vi "Advanced Params.vi"(6 "ID (Profile)":string="Profile", 7 "ADV params":T1={"ID"="", "Units"=enum."Metric", "RefPos"=0.0, "Cycles"=1, "Steps"=1, "Autoreturn"=FALSE, "BreakStop"=FALSE} {"Steps" min=1 max=12 step=1; "Cycles" min=1 max=60000 step=1}, 8 "error in (no error)":errorcluster, 11 "Profile NO":u8=1 min=1 max=50 step=1) -> (0 "error out":errorcluster, 2 "wchitch params":string, 3 "params array out":string[](array[string]))   [LabVIEW 2019, in "STAV lib.lvlib"]
uses:
  STAV lib.lvlib
  Advanced prams.ctl
  Param Units.ctl
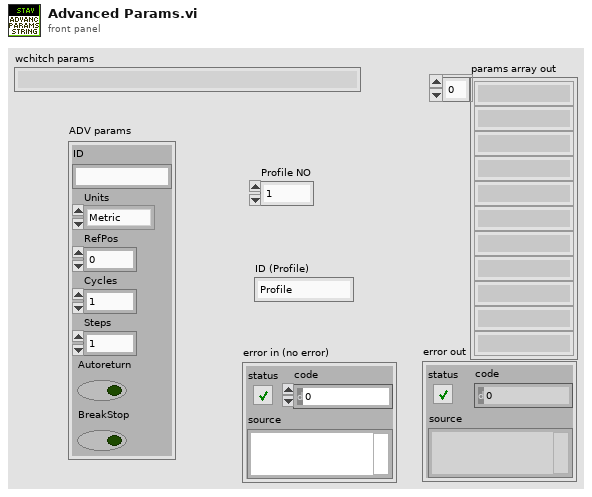
[diagram p1: front panel]
types:
  T1 = typedef "STAV lib.lvlib/Advanced prams.ctl" = cluster{"ID":string, "Units":T2, "RefPos":dbl, "Cycles":i32, "Steps":i32, "Autoreturn":bool, "BreakStop":bool}
  T2 = typedef "STAV lib.lvlib/Param Units.ctl" = enum16{"Metric", "Imperial"}
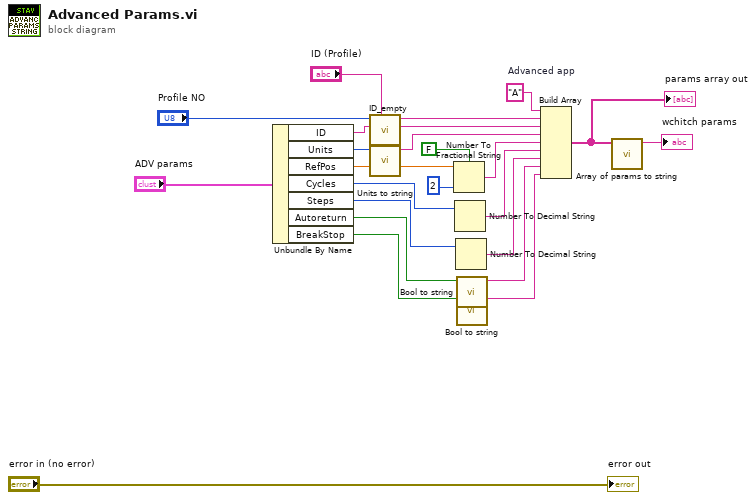
[diagram p0: block diagram]
diagram:
  w24 = "A"  # Advanced app
  n1 = Unbundle By Name("ADV params") -> ("ID"=w14:string, "Units"=w21:T2, "RefPos"=w20:dbl, "Cycles"=w8:i32, "Steps"=w7:i32, "Autoreturn"=w6:bool, "BreakStop"=w5:bool)
  n2 = call "ID_empty.vi"("ID (Profile)"="ID (Profile)", "ID in"=w14, "Profile NO"="Profile NO") -> ("ID out"=w13:string, "Profile NO out"=w15:string)  [unwired: 7 in]
  n3 = call "Units to string.vi"("Units"=w21) -> ("Peak app"=w19:string)  [unwired: 10 in]
  n4 = Number To Fractional String(use system decimal point (T)=FALSE, number=w20, precision (6)=i16 2) -> (F-format string=w18:string)  [unwired: 1 in]
  n5 = Number To Decimal String(number=w8) -> (decimal integer string=w4:string)  [unwired: 1 in]
  n6 = Number To Decimal String(number=w7) -> (decimal integer string=w3:string)  [unwired: 1 in]
  n7 = call "Bool to string.vi"("Autoreturn"=w6) -> ("Peak app"=w2:string)  [unwired: 10 in]
  n8 = call "Bool to string.vi"("Autoreturn"=w5) -> ("Peak app"=w1:string)  [unwired: 10 in]
  n9 = Build Array(w24, w15, w13, w19, w18, w4, w3, w2, w1) -> (w12:string[])
  "params array out" <- w12
  n10 = call "Array of params to string.vi"("Array"=w12) -> ("String"=→"wchitch params":string)  [unwired: 10 in]
  "error out" <- "error in (no error)"
